vi "Send Handle Last Ack.vi"(9 "Error Report":errorcluster, 10 "State":variant, 11 "Ident":string) -> (2 "channel out":T1)   [LabVIEW 2019, in "Cmd-Data Event Messages.lvlib"]
uses:
  Cmd-Data Event Messages.lvlib
  template/Last Ack.ctl
  cmd-data event messenger/source/Cmd-Data Event Messenger.lvlib
  cmd-data event messenger/source/))Channel.ctl
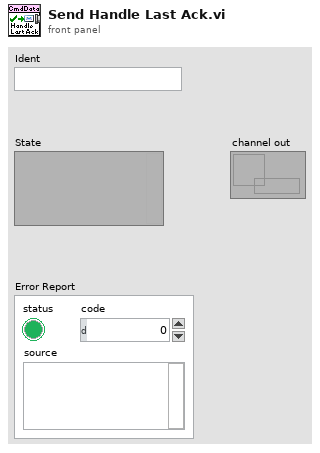
[diagram p1: front panel]
types:
  T1 = typedef "Cmd-Data Event Messenger.lvlib/))Channel.ctl" = refnum<queue>
  T2 = typedef "Cmd-Data Event Messages.lvlib/Last Ack.ctl" = cluster{"Ident":string, "Error Report":errorcluster, "State ":string}
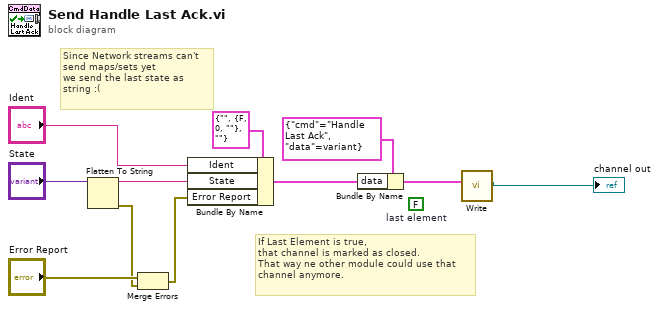
[diagram p0: block diagram]
diagram:
  (unwired) FALSE  # last element
  # "If Last Element is true,\nthat channel is marked as closed.\nThat way ne other module could use that\nchannel anymore."
  # "Since Network streams can't\nsend maps/sets yet\nwe send the last state as\nstring :("
  n1 = Flatten To String(anything="State") -> (data string=w5:string, error out=w3:errorcluster)  [unwired: 3 in, 1 out]
  n2 = Merge Errors("Error Report", w3) -> (w4:errorcluster)
  n3 = Bundle By Name(cluster=T2 {"Ident"="", "Error Report"={"status"=FALSE, "code"=0, "source"=""}, "State "=""} ("Last Ack"), "Ident"="Ident", "State"=w5, "Error Report"=w4) -> (w11:T2)
  n4 = Bundle By Name(cluster=cluster{"cmd":string, "data":variant} {"cmd"="Handle Last Ack", "data"=variant} ("message"), "data"=w11) -> (w2:cluster{"cmd":string, "data":variant})
  n5 = call "Write.vi"("element"=w2) -> ("channel out"=→"channel out":T1)  [unwired: 9 in, 1 out]
